vi "Write NET_HttpContentHeaders.vi"(8 "error in (no error)":errorcluster, 10 "HttpContentHeaders":refnum<k24>, 11 "HttpHeaders_Request in":refnum<class "HttpHeaders_Content.lvclass">) -> (0 "error out":errorcluster, 3 "HttpHeaders_Request out":refnum<class "HttpHeaders_Content.lvclass">)   [LabVIEW 2018, in "HttpClient_NET.lvlib" / "HttpHeaders_Content.lvclass"]
uses:
  HttpHeaders_Content.lvclass
  C:/Viviota/Projects/R&D/LabVIEW_HTTP_REST_NET/HTTPHeaders_NET/HttpHeaders_NET.lvclass
  System.Net.Http
  HTTPHeaders_NET/HttpHeaders_NET.lvclass/HttpHeaders_NET.ctl
  HTTPHeaders_NET/HttpHeaders_NET.lvclass
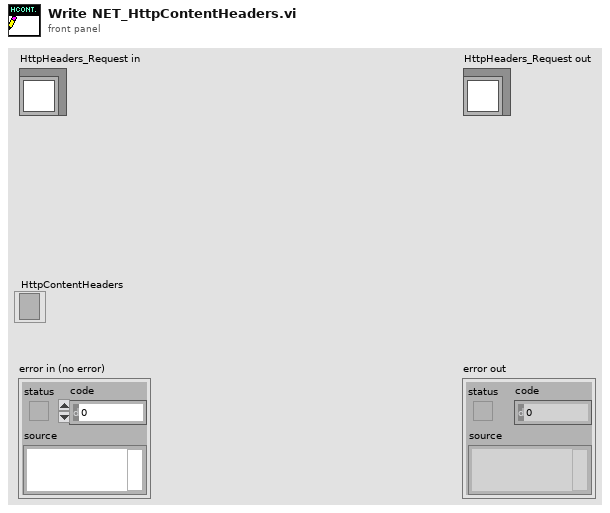
[diagram p1: front panel]
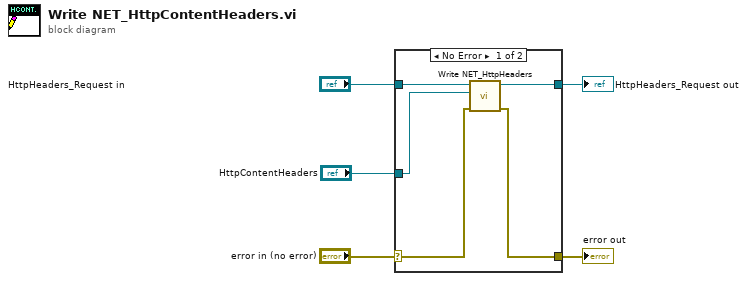
[diagram p0: block diagram]
diagram:
  n1 = case shown="No Error" "error in (no error)" {
    selector: "error in (no error)" -> [w7 w11]
    tunnel: [w6 w11] -> w4
    tunnel: [w9 w12] -> w2
    tunnel: "HttpHeaders_Request in" -> [w10 w12]
    tunnel: "HttpContentHeaders" -> [w8 _]
    frame No Error {
      n2 = call "Write NET_HttpHeaders.vi"("error in (no error)"=w7, "NET_HttpHeaders"=w8, "HTTPHeaders_NET in"=w10) -> ("error out"=w6:errorcluster, "HTTPHeaders_NET out"=w9:refnum<class "HttpHeaders_Content.lvclass">)  [unwired: 7 in]
    }
    frame Error {
    }
  }
  "error out" <- w4
  "HttpHeaders_Request out" <- w2
